vi "Find Mid Point (SubVI).vi"(10 "Point 2":u32, 11 "Point 1":u32) -> (0 "Mid Point (Int)":u32, 3 "Mid Point":u32)   [LabVIEW 2015]
uses:
  <vilib>/rvi/FXPMathLib/FxpDiv/subVIs/nifxpmath_Div_SimConfig.ctl
  <vilib>/rvi/FXPMathLib/FxpDiv/simVIs/DllFxpDivTemp_sub.vi
  <vilib>/rvi/FXPMathLib/FxpDiv/XNode/nifxpmath_Div.xnode
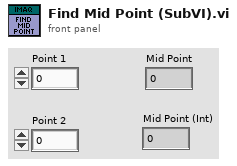
[diagram p1: front panel]
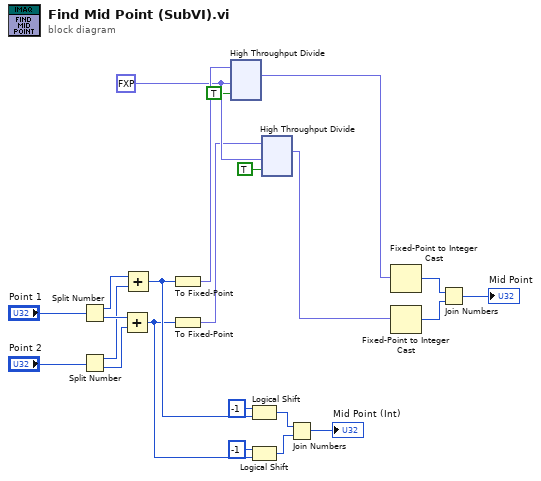
[diagram p0: block diagram]
diagram:
  w5 = fxp<+,2,2> 2.0 ("y")
  n1 = Split Number(x="Point 1") -> (hi(x)=w17:u16, lo(x)=w19:u16)
  n2 = Split Number(x="Point 2") -> (hi(x)=w18:u16, lo(x)=w20:u16)
  n3 = Add(x=w19, y=w20) -> (x+y=w11:u16)
  n4 = Add(x=w17, y=w18) -> (x+y=w12:u16)
  n5 = To Fixed-Point(number=w12) -> (fixed-point=w6:fxp<+,16,9>)  [unwired: 1 in]
  n6 = To Fixed-Point(number=w11) -> (fixed-point=w1:fxp<+,16,9>)  [unwired: 1 in]
  n7 = xnode "High Throughput Divide"("x"=w6, "y"=w5, "input valid"=TRUE) -> ("x/y"=w7:fxp<+,16,9>)  [unwired: 1 in, 2 out]
  n8 = Logical Shift(y=i16 -1, x=w12) -> (x << y=w9:u16)
  n9 = Logical Shift(y=i16 -1, x=w11) -> (x << y=w10:u16)
  n10 = xnode "High Throughput Divide"("x"=w1, "y"=w5, "input valid"=TRUE) -> ("x/y"=w4:fxp<+,16,9>)  [unwired: 1 in, 2 out]
  n11 = Join Numbers(hi=w9, lo=w10) -> ((hi.lo)=→"Mid Point (Int)":u32)
  n12 = Fixed-Point to Integer Cast(1:w7) -> (0:w16:u16)
  n13 = Fixed-Point to Integer Cast(1:w4) -> (0:w15:u16)
  n14 = Join Numbers(hi=w16, lo=w15) -> ((hi.lo)=→"Mid Point":u32)
